vi "CRYAuto Save DB.vi"(0 "Setup in":T1={"No.VI"=0, "Category"="", "StepName"="", "Seq setup flattened"="", "Comment"="", "Steps config."=[], "Jump config"=[], "Start"=0.0, "Increment"=0.0, "Name"="Pa", "Unit"="Pa", "Y data"=1, "Y prefix"="", "Y dB ref"=1.0, "Y unit"="", "Repeat State Array"=[]} {"Repeat State Array"."Start" format="%#_5g"; "Y dB ref" format="%.1f"; "Y data" items=["dB", "Lin"]; "Start" format="%#_5g"}) -> ()   [LabVIEW 2013]
uses:
  Typedef Control/CRYStep.ctl
  Data/CRYData & result stacks global.vi
  CRYMainGlobal.vi
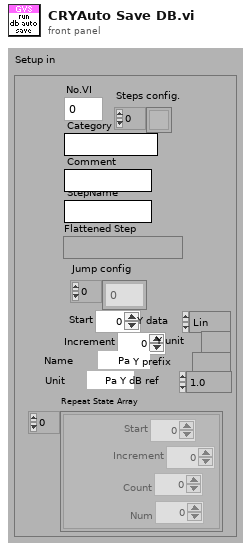
[diagram p1: front panel]
types:
  T1 = typedef "CRYStep.ctl" = cluster{"No.VI":i32, "Category":string, "StepName":string, "Seq setup flattened":string, "Comment":string, "Steps config.":bool[], "Jump config":i32[], "Start":dbl, "Increment":dbl, "Name":string, "Unit":string, "Y data":u16, "Y prefix":string, "Y dB ref":dbl, "Y unit":string, "Repeat State Array":cluster{"Start":dbl, "Increment":dbl, "Count":i32, "Num":i32}[]}
  T2 = enum16{"OK", "Yes", "YesNo", "YesNoCancel", "ReplaceAppend"}
  T3 = cluster{"Curve_ID":u32, "Datarun_ID":i32, "Number_of_Points":i32, "Channel_Type_ID":i32, "Axis_ID":i32, "Curve_Type_ID":i32, "Verdict_ID":i32, "Unit_ID":i32}
  T4 = typedef "CRYAuto Save Cluster.ctl" = cluster{"Name":string, "save":enum16{"Data", "Results", "Waveforms"}, "Item Names":string[], "Autosave folder":path, "data format":u16, "filename option":enum16{"auto", "prompt"}, "fn construction":i32[], "layout":enum16{"rows", "columns"}, "notation":enum16{"sci", "float"}, "precision":i32, "prompt comment":bool, "header":enum16{"none", "standard", "custom"}, "custom header":string, "serial no.":bool, "User defined":string, "delimiter":enum16{"tab", "comma", "space", "other"}, "other delim":string, "axes":cluster{"x":bool, "y":bool, "z":bool}, "Time Stamp":bool, "Lot No.":bool, "Operator":bool, "Excel Template":string, "New or Append":u16, "Data":u16, "Help":string, "Tab Value":enum32{"Setting", "Help"}, "UDL or DSN":path, "User Default":bool, "Selector":i32, "Axis":u16, "Value Name":string, "format string":cluster{"dB Format String out":string, "Lin Format String out":string}, "DBPath":path}
  T5 = typedef "NI_Database_API.lvlib/Conn ObjectReference.ctl" = refnum<k1>
  T6 = typedef "CRYData Cluster Array.ctl" = T7[]
  T7 = typedef "CRYData Cluster.ctl" = cluster{"Name":string, "Curve":cluster{"x":dbl, "y":dbl, "z":dbl}[], "X data":u16, "Y data":u16, "Z data":u16, "X axis":u16, "Y axis":u16, "Z axis":u16, "X unit":string, "Y unit":string, "Z unit":string, "X dB ref":dbl, "Y dB ref":dbl, "Z dB ref":dbl, "single val":bool, "protected":bool, "display X":bool, "display Y":bool, "display Z":bool, "Test Info":string, "Step No.":i32, "Plot Settings":cluster{"Color":u32, "Interpolation":u8, "Point Style":u8, "Line Style":u8, "Point Color":u32, "Line Width":u8, "Bar Plot Style":u8, "Fill To":i16}, "AutoProtect":bool}
  T8 = typedef "CRYResult Cluster Array.ctl" = T9[]
  T9 = typedef "CRYResult Cluster.ctl" = cluster{"Name":string, "Margin":dbl, "unit":string, "Verdict":bool, "Limit":string, "Max/Min":string, "protected":bool, "Step No.":i32, "Test Info":string, "AutoProtect":bool}
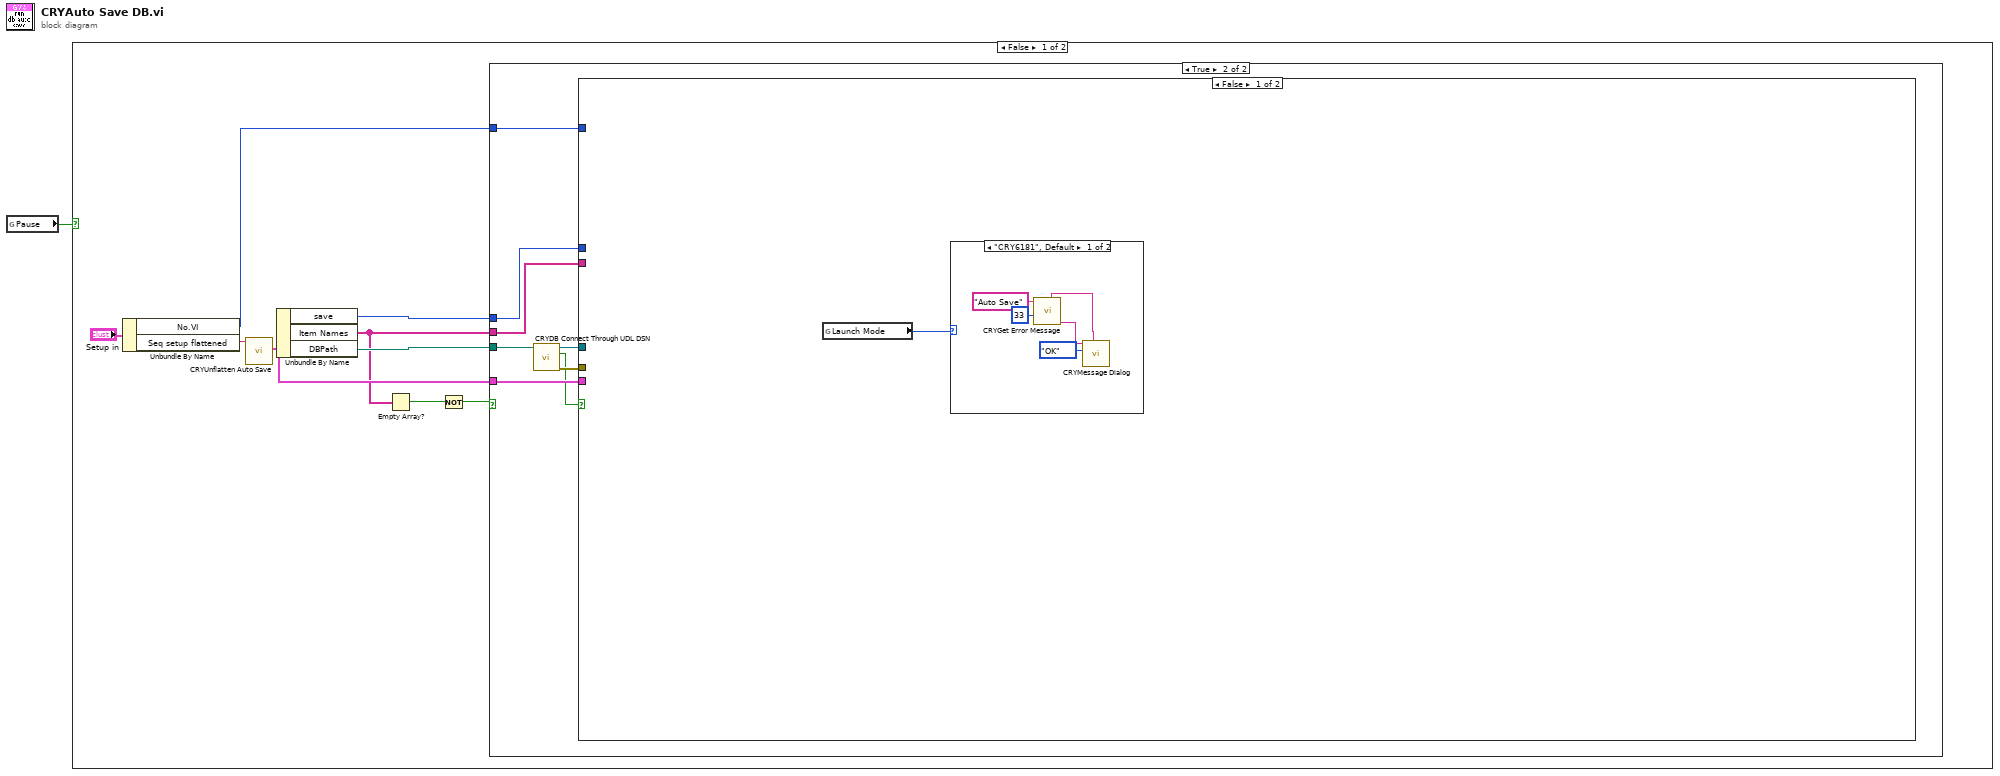
[diagram p0: block diagram]
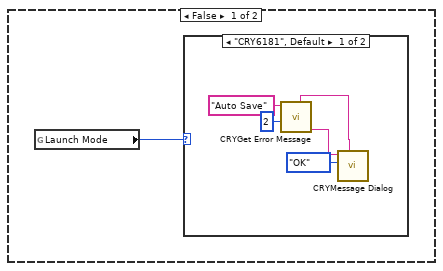
[diagram p2: hidden frame]
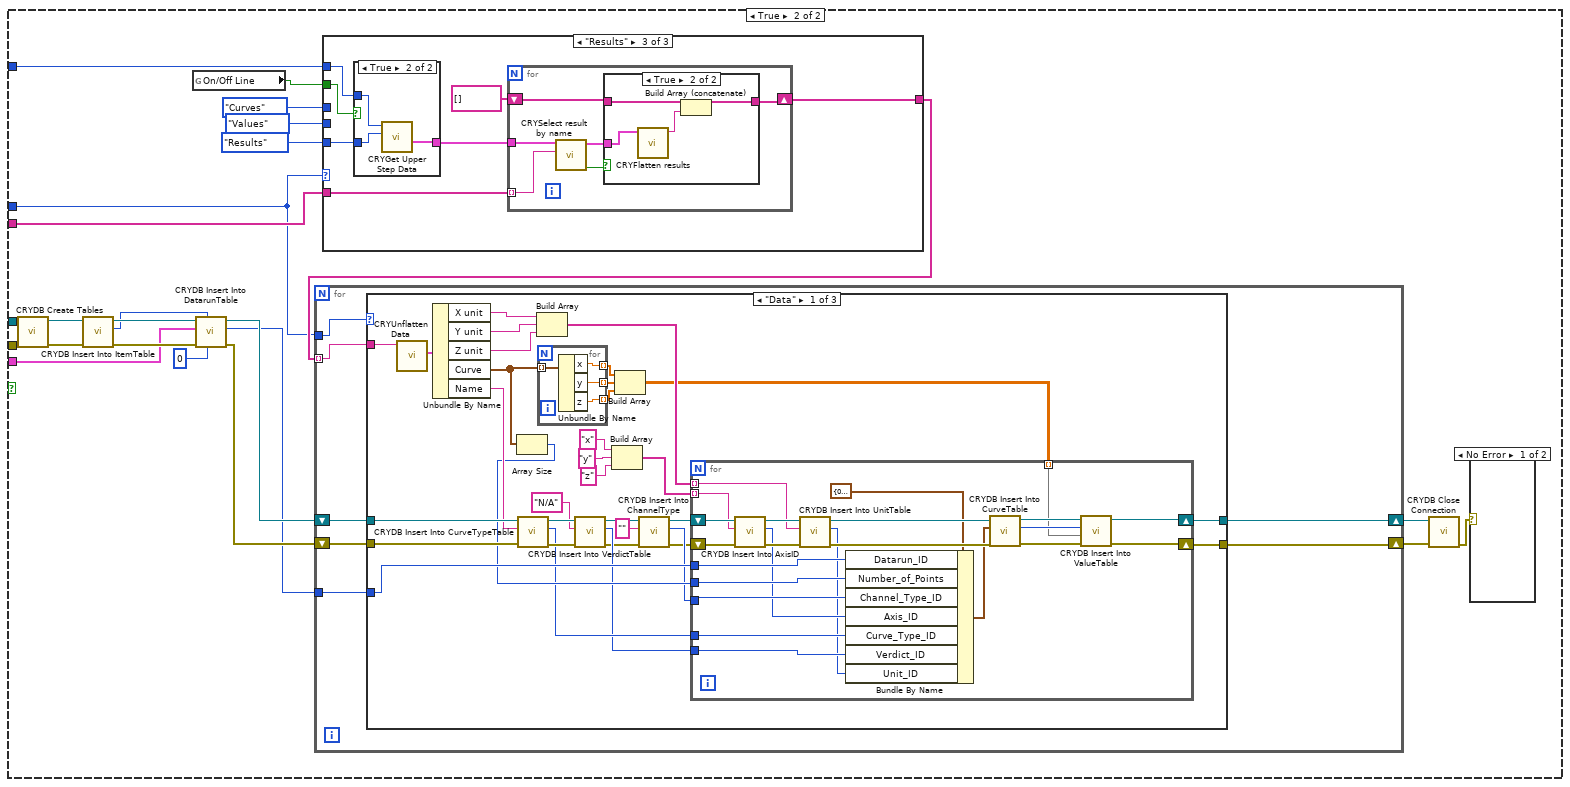
[diagram p5: hidden frame]
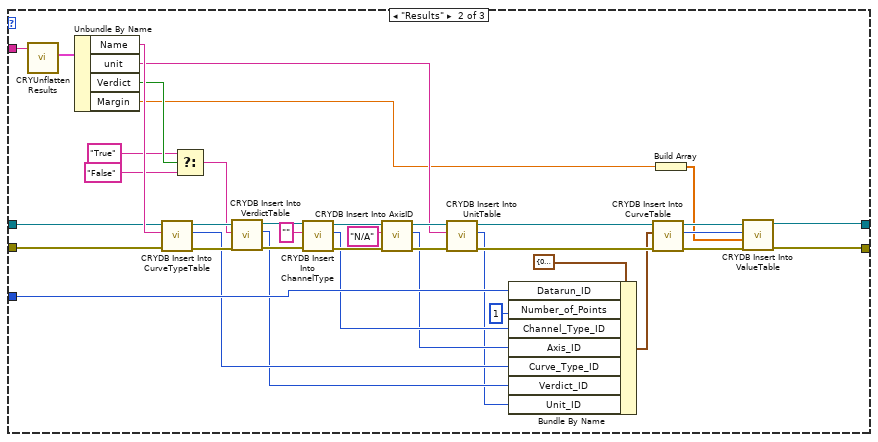
[diagram p7: hidden frame]
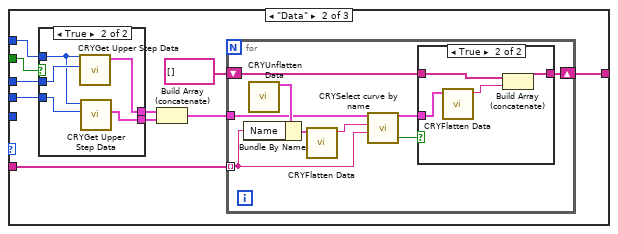
[diagram p10: hidden frame]
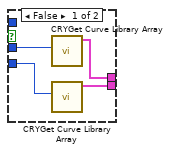
[diagram p11: hidden frame]
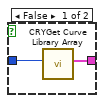
[diagram p13: hidden frame]
diagram:
  n1 = global read "CRYData & result stacks global.vi" "Pause"() -> (w1:bool)
  n2 = case shown="False" w1 {
    frame False {
      n3 = Unbundle By Name("Setup in") -> ("No.VI"=w6:i32, "Seq setup flattened"=w9:string)
      n4 = call "CRYUnflatten Auto Save.vi"("Flatten Auto Save"=w9) -> ("Auto save"=w7:T4)  [unwired: 8 in, 2 out]
      n5 = Unbundle By Name(w7) -> ("save"=w5:enum16{"Data", "Results", "Waveforms"}, "Item Names"=w4:string[], "DBPath"=w8:path)
      n6 = Empty Array?(array=w4) -> (empty?=w3:bool)
      n7 = Not(x=w3) -> (.not. x?=w2:bool)
      n8 = case shown="True" w2 {
        tunnel: w8 -> [_ w24]
        tunnel: w7 -> [_ w21]
        tunnel: w6 -> [_ w20]
        tunnel: w4 -> [_ w19]
        tunnel: w5 -> [_ w18]
        frame False {
          n9 = global read "CRYMainGlobal.vi" "Launch Mode"() -> (w11:enum32{"CRY6181", "CRY6181 One"})
          n10 = case shown="\"CRY6181\", Default" w11 {
            frame "CRY6181", Default {
              n11 = call "CRYGet Error Message.vi"("Error No"=2, "Kind"="Auto Save") -> ("Message Sub 3"=w15:string, "Window Title"=w13:string)  [unwired: 4 in, 4 out]
              n12 = call "CRYMessage Dialog.vi"("Window Title"=w13, "YesNoCancel"=T2."OK", "Message Content"=w15) -> ()  [unwired: 7 in, 2 out]
            }
            frame "CRY6181 One" {
            }
          }
        }
        frame True {
          n13 = call "CRYDB Connect Through UDL DSN.vi"("DB Path"=w24) -> ("error out"=w22:errorcluster, "bResult"=w17:bool, "connection reference"=w23:T5)  [unwired: 8 in]
          n14 = case shown="False" w17 {
            tunnel: w23 -> [_ w53]
            tunnel: w22 -> [_ w52]
            tunnel: w21 -> [_ w45]
            tunnel: w20 -> [_ w41]
            tunnel: w19 -> [_ w33]
            tunnel: w18 -> [_ w32]
            frame False {
              n15 = global read "CRYMainGlobal.vi" "Launch Mode"() -> (w25:enum32{"CRY6181", "CRY6181 One"})
              n16 = case shown="\"CRY6181\", Default" w25 {
                frame "CRY6181", Default {
                  n17 = call "CRYGet Error Message.vi"("Error No"=33, "Kind"="Auto Save") -> ("Message Sub 3"=w29:string, "Window Title"=w27:string)  [unwired: 4 in, 4 out]
                  n18 = call "CRYMessage Dialog.vi"("Window Title"=w27, "YesNoCancel"=T2."OK", "Message Content"=w29) -> ()  [unwired: 7 in, 2 out]
                }
                frame "CRY6181 One" {
                }
              }
            }
            frame True {
              n19 = call "CRYDB Create Tables.vi"("error in"=w52, "connection reference"=w53) -> ("error out"=w51:errorcluster, "connection reference out"=w50:T5)  [unwired: 8 in]
              n20 = call "CRYDB Insert Into ItemTable.vi"("connection reference"=w50, "error in"=w51) -> ("connection reference out"=w49:T5, "Item_ID"=w47:i32, "error out"=w48:errorcluster)  [unwired: 6 in]
              n21 = global read "CRYMainGlobal.vi" "On/Off Line"() -> (w40:bool)
              n22 = call "CRYDB Insert Into DatarunTable.vi"("Station_ID"=0, "Item_ID"=w47, "error in"=w48, "Auto save"=w45, "connection reference"=w49) -> ("error out"=w38:errorcluster, "Datarun_ID"=w36:i32, "connection reference out"=w39:T5)  [unwired: 4 in]
              n23 = case shown="\"Results\"" w32 {
                tunnel: w33 -> [_ w171 w198]
                tunnel: [string[] [] w170 w201] -> w37
                tunnel: enum16{"Curves", "Values", "Results", "WFM"}."Curves" ("Type") -> [_ w169 _]
                tunnel: enum16{"Curves", "Values", "Results", "WFM"}."Values" ("Type") -> [_ w168 _]
                tunnel: enum16{"Curves", "Values", "Results", "WFM"}."Results" ("Type") -> [_ _ w200]
                tunnel: w41 -> [_ w163 w196]
                tunnel: w40 -> [_ w164 w197]
                frame Default {
                }
                frame "Data" {
                  n24 = case shown="True" w164 {
                    tunnel: w169 -> [w175 w180]
                    tunnel: w168 -> [w174 w179]
                    tunnel: [w173 w177] -> w167
                    tunnel: [w172 w176] -> w165
                    tunnel: w163 -> [_ w178]
                    frame False {
                      n25 = call "CRYGet Curve Library Array.vi"("Type In"=w175) -> ("Curve/Value array"=w173:T6)  [unwired: 10 out]
                      n26 = call "CRYGet Curve Library Array.vi"("Type In"=w174) -> ("Curve/Value array"=w172:T6)  [unwired: 10 out]
                    }
                    frame True {
                      n27 = call "CRYGet Upper Step Data.vi"("Type In"=w180, "No.VI"=w178) -> ("Curve array"=w177:T6)  [unwired: 9 out]
                      n28 = call "CRYGet Upper Step Data.vi"("Type In"=w179, "No.VI"=w178) -> ("Value array"=w176:T6)  [unwired: 9 out]
                    }
                  }
                  n29 = Build Array (concatenate)(w167, w165) -> (w166:T6)
                  n30 = for {
                    tunnel: w166 -> [w182]
                    tunnel: w171 -> [w181] mode=indexing
                    shift-right: [w185] -> w170
                    shift-left: string[] [] -> [w186]
                    n31 = call "CRYUnflatten Data.vi"() -> ("Datum"=w188:T7)  [unwired: 9 in, 2 out]
                    n32 = Bundle By Name(cluster=w188, "Name"=w181) -> (w189:T7)
                    n33 = call "CRYFlatten Data.vi"("Datum"=w189) -> ("Data flattened"=w187:string)  [unwired: 10 in]
                    n34 = call "CRYSelect curve by name.vi"("Curve name desired (just name, if flat data not wired)"=w181, "Curve name desired (flat data)"=w187, "Data array"=w182) -> ("Exists?"=w184:bool, "Desired Curve"=w183:T7)  [unwired: 5 in, 2 out]
                    n35 = case shown="True" w184 {
                      tunnel: w186 -> [w190 w194]
                      tunnel: [w190 w193] -> w185
                      tunnel: w183 -> [_ w191]
                      frame False {
                      }
                      frame True {
                        n36 = call "CRYFlatten Data.vi"("Datum"=w191) -> ("Data flattened"=w192:string)  [unwired: 10 in]
                        n37 = Build Array (concatenate)(w194, w192) -> (w193:string[])
                      }
                    }
                  }
                }
                frame "Results" {
                  n38 = case shown="True" w197 {
                    tunnel: w200 -> [w203 w206]
                    tunnel: [w202 w204] -> w199
                    tunnel: w196 -> [_ w205]
                    frame False {
                      n39 = call "CRYGet Curve Library Array.vi"("Type In"=w203) -> ("Result array"=w202:T8)  [unwired: 10 out]
                    }
                    frame True {
                      n40 = call "CRYGet Upper Step Data.vi"("Type In"=w206, "No.VI"=w205) -> ("Result array"=w204:T8)  [unwired: 9 out]
                    }
                  }
                  n41 = for {
                    tunnel: w199 -> [w207]
                    tunnel: w198 -> [w212] mode=indexing
                    shift-right: [w210] -> w201
                    shift-left: string[] [] -> [w211]
                    n42 = call "CRYSelect result by name.vi"("Result name desired"=w212, "Result array"=w207) -> ("Exists?"=w208:bool, "Desired Result"=w209:T9)  [unwired: 8 in]
                    n43 = case shown="True" w208 {
                      tunnel: w211 -> [w213 w217]
                      tunnel: [w213 w216] -> w210
                      tunnel: w209 -> [_ w214]
                      frame False {
                      }
                      frame True {
                        n44 = call "CRYFlatten results.vi"("Result in"=w214) -> ("Flatten Result"=w215:string)  [unwired: 10 in]
                        n45 = Build Array (concatenate)(w217, w215) -> (w216:string[])
                      }
                    }
                  }
                }
              }
              n46 = for {
                tunnel: w37 -> [w58] mode=indexing
                shift-right: [w55] -> w34
                shift-left: w39 -> [w60]
                shift-right: [w54] -> w35
                shift-left: w38 -> [w59]
                tunnel: w32 -> [w57]
                tunnel: w36 -> [w56]
                n47 = case shown="\"Data\"" w57 {
                  tunnel: w60 -> [w93 w155 w160]
                  tunnel: w59 -> [w92 w154 w159]
                  tunnel: w58 -> [w90 w158 _]
                  tunnel: w56 -> [w71 w134 _]
                  tunnel: [w64 w124 w160] -> w55
                  tunnel: [w63 w123 w159] -> w54
                  frame "Data" {
                    n48 = call "CRYUnflatten Data.vi"("Unflatten data"=w90) -> ("Datum"=w89:T7)  [unwired: 8 in, 2 out]
                    n49 = Unbundle By Name(w89) -> ("X unit"=w87:string, "Y unit"=w86:string, "Z unit"=w85:string, "Curve"=w70:cluster{"x":dbl, "y":dbl, "z":dbl}[], "Name"=w88:string)
                    n50 = Array Size(array=w70) -> (size(s)=w69:i32)
                    n51 = call "CRYDB Insert Into CurveTypeTable.vi"("connection reference"=w93, "Curve Name"=w88, "error in"=w92) -> ("connection reference out"=w91:T5, "Curve_Type_ID"=w67:i32, "error out"=w83:errorcluster)  [unwired: 5 in]
                    n52 = Build Array(w87, w86, w85) -> (w78:string[])
                    n53 = for {
                      tunnel: w70 -> [w120] mode=indexing
                      tunnel: [w119] -> w81 mode=indexing
                      tunnel: [w118] -> w80 mode=indexing
                      tunnel: [w117] -> w79 mode=indexing
                      n54 = Unbundle By Name(w120) -> ("x"=w119:dbl, "y"=w118:dbl, "z"=w117:dbl)
                    }
                    n55 = call "CRYDB Insert Into VerdictTable.vi"("connection reference"=w91, "Veridict Name"="N/A", "error in"=w83) -> ("connection reference out"=w84:T5, "Verdict_ID"=w66:i32, "error out"=w62:errorcluster)  [unwired: 5 in]
                    n56 = Build Array("x" ("Veridict Name"), "y" ("Veridict Name"), "z" ("Veridict Name")) -> (w74:string[])
                    n57 = Build Array(w81, w80, w79) -> (w65:dbl[][])
                    n58 = call "CRYDB Insert Into ChannelType.vi"("connection reference"=w84, "Channel Type Name"="", "error in"=w62) -> ("connection reference out"=w73:T5, "Channel_Type_ID"=w68:i32, "error out"=w61:errorcluster)  [unwired: 5 in]
                    n59 = for {
                      tunnel: w78 -> [w111] mode=indexing
                      shift-right: [w98] -> w64
                      shift-left: w73 -> [w116]
                      shift-right: [w94] -> w63
                      shift-left: w61 -> [w115]
                      tunnel: w74 -> [w114] mode=indexing
                      tunnel: w71 -> [w107]
                      tunnel: w69 -> [w106]
                      tunnel: w68 -> [w105]
                      tunnel: w67 -> [w103]
                      tunnel: w66 -> [w102]
                      tunnel: w65 -> [w96] mode=indexing
                      n60 = call "CRYDB Insert Into AxisID.vi"("connection reference"=w116, "Axies Name"=w114, "error in"=w115) -> ("connection reference out"=w113:T5, "Axis_ID"=w104:i32, "error out"=w112:errorcluster)  [unwired: 5 in]
                      n61 = call "CRYDB Insert Into UnitTable.vi"("connection reference"=w113, "Unit_Abbreviation"=w111, "error in"=w112) -> ("connection reference out"=w110:T5, "Unit ID"=w101:i32, "error out"=w109:errorcluster)  [unwired: 5 in]
                      n62 = Bundle By Name(cluster=T3 {"Curve_ID"=0, "Datarun_ID"=0, "Number_of_Points"=0, "Channel_Type_ID"=0, "Axis_ID"=0, "Curve_Type_ID"=0, "Verdict_ID"=0, "Unit_ID"=0} ("Curve_Table Data"), "Datarun_ID"=w107, "Number_of_Points"=w106, "Channel_Type_ID"=w105, "Axis_ID"=w104, "Curve_Type_ID"=w103, "Verdict_ID"=w102, "Unit_ID"=w101) -> (w100:T3)
                      n63 = call "CRYDB Insert Into CurveTable .vi"("error in"=w109, "Curve_Table Data"=w100, "connection reference"=w110) -> ("error out"=w95:errorcluster, "Curve ID"=w97:i32, "connection reference out"=w99:T5)  [unwired: 6 in]
                      n64 = call "CRYDB Insert Into ValueTable.vi"("connection reference"=w99, "Curve_ID"=w97, "Value"=w96, "error in"=w95) -> ("connection reference out"=w98:T5, "error out"=w94:errorcluster)  [unwired: 5 in]
                    }
                  }
                  frame "Results" {
                    n65 = call "CRYUnflatten Results.vi"("Unflatten Result"=w158) -> ("Result"=w157:T9)  [unwired: 8 in, 2 out]
                    n66 = Unbundle By Name(w157) -> ("Name"=w156:string, "unit"=w139:string, "Verdict"=w152:bool, "Margin"=w122:dbl)
                    n67 = call "CRYDB Insert Into CurveTypeTable.vi"("connection reference"=w155, "Curve Name"=w156, "error in"=w154) -> ("connection reference out"=w153:T5, "Curve_Type_ID"=w130:i32, "error out"=w148:errorcluster)  [unwired: 5 in]
                    n68 = Select(t="True" ("Name"), s=w152, f="False" ("Name")) -> (s? t:f=w149:string)
                    n69 = call "CRYDB Insert Into VerdictTable.vi"("connection reference"=w153, "Veridict Name"=w149, "error in"=w148) -> ("connection reference out"=w147:T5, "Verdict_ID"=w129:i32, "error out"=w142:errorcluster)  [unwired: 5 in]
                    n70 = call "CRYDB Insert Into ChannelType.vi"("connection reference"=w147, "Channel Type Name"="", "error in"=w142) -> ("connection reference out"=w145:T5, "Channel_Type_ID"=w132:i32, "error out"=w143:errorcluster)  [unwired: 5 in]
                    n71 = call "CRYDB Insert Into AxisID.vi"("connection reference"=w145, "Axies Name"="N/A", "error in"=w143) -> ("connection reference out"=w144:T5, "Axis_ID"=w131:i32, "error out"=w140:errorcluster)  [unwired: 5 in]
                    n72 = call "CRYDB Insert Into UnitTable.vi"("connection reference"=w144, "Unit_Abbreviation"=w139, "error in"=w140) -> ("connection reference out"=w137:T5, "Unit ID"=w128:i32, "error out"=w136:errorcluster)  [unwired: 5 in]
                    n73 = Bundle By Name(cluster=T3 {"Curve_ID"=0, "Datarun_ID"=0, "Number_of_Points"=0, "Channel_Type_ID"=0, "Axis_ID"=0, "Curve_Type_ID"=0, "Verdict_ID"=0, "Unit_ID"=0} ("Curve_Table Data"), "Datarun_ID"=w134, "Number_of_Points"=1, "Channel_Type_ID"=w132, "Axis_ID"=w131, "Curve_Type_ID"=w130, "Verdict_ID"=w129, "Unit_ID"=w128) -> (w135:T3)
                    n74 = call "CRYDB Insert Into CurveTable .vi"("error in"=w136, "Curve_Table Data"=w135, "connection reference"=w137) -> ("error out"=w125:errorcluster, "Curve ID"=w126:i32, "connection reference out"=w127:T5)  [unwired: 6 in]
                    n75 = Build Array(w122) -> (w121:dbl[])
                    n76 = call "CRYDB Insert Into ValueTable.vi"("connection reference"=w127, "Curve_ID"=w126, "Value"=w121, "error in"=w125) -> ("connection reference out"=w124:T5, "error out"=w123:errorcluster)  [unwired: 5 in]
                  }
                  frame Default {
                  }
                }
              }
              n77 = call "CRYDB Close Connection.vi"("error in"=w35, "connection reference"=w34) -> ("error out"=w31:errorcluster)  [unwired: 9 in]
              n78 = case shown="No Error" w31 {
                frame No Error {
                }
                frame Error {
                }
              }
            }
          }
        }
      }
    }
    frame True {
    }
  }
